vi "_Read.vi"(8 "error in (no error)":errorcluster, 11 "Photon Counter SR400 in":refnum<class "Photon Counter SR400.lvclass">) -> (0 "error out":errorcluster, 2 "4 Data Points":dbl[](array[numeric]), 3 "Photon Counter SR400 out":refnum<class "Photon Counter SR400.lvclass">)   [LabVIEW 2015, in "Photon Counter SR400.lvclass"]
uses:
  Photon Counter SR400.lvclass
  SR400/SR400.lvlib
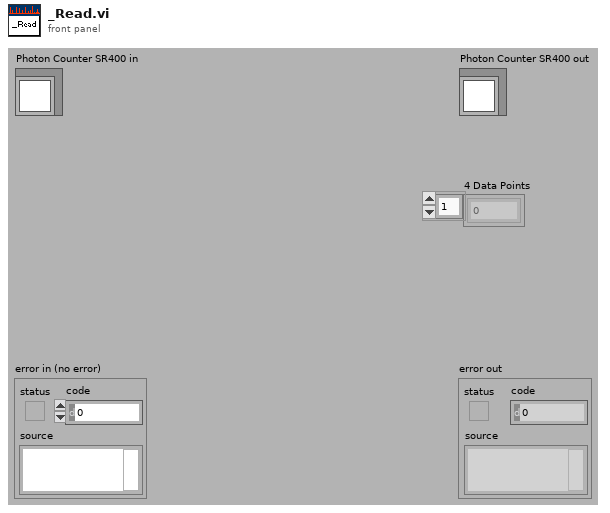
[diagram p1: front panel]
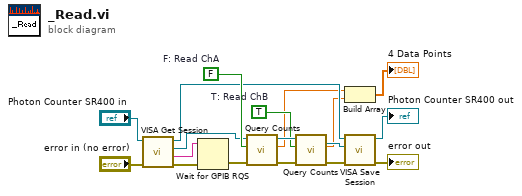
[diagram p0: block diagram]
diagram:
  w13 = TRUE  # T: Read ChB
  w14 = FALSE  # F: Read ChA
  n1 = call-dynamic "VISA Get Session.vi"("error in (no error)"="error in (no error)", "Instrument.lvclass in"="Photon Counter SR400 in") -> ("error out"=w8:errorcluster, "GPIB string"=w2:string, "VISA Resource Name"=w1:refnum<visa-resource-name>, "Instrument.lvclass out"=w11:refnum<class "Photon Counter SR400.lvclass">)  [unwired: 6 out]
  n2 = Wait for GPIB RQS(2:w8, 4:w2) -> (0:w12:errorcluster)  [unwired: 1 in, 1 out]
  n3 = call "Query Counts.vi"("error in (no error)"=w12, "Read B?"=w14, "VISA resource name"=w1) -> ("error out"=w17:errorcluster, "Counts"=w7:dbl, "VISA resource name out"=w18:refnum<visa-resource-name>)  [unwired: 6 out]
  n4 = call "Query Counts.vi"("error in (no error)"=w17, "Read B?"=w13, "VISA resource name"=w18) -> ("error out"=w16:errorcluster, "Counts"=w6:dbl, "VISA resource name out"=w15:refnum<visa-resource-name>)  [unwired: 6 out]
  n5 = Build Array(w7, w6) -> (→"4 Data Points":dbl[])
  n6 = call-dynamic "VISA Save Session.vi"("error in (no error)"=w16, "VISA Resource Name"=w15, "Instrument.lvclass in"=w11) -> ("error out"=→"error out":errorcluster, "Instrument.lvclass out"=→"Photon Counter SR400 out":refnum<class "Photon Counter SR400.lvclass">)  [unwired: 7 out]
